vi "LockinFrontPanel.vi"() -> ()   [LabVIEW 2021]
panel:
  in  "?":enum32{"Main", "Phase", "Misc", "Stop"}(tab)
  in  "Set Amplitude":dbl
  in  "Set Amp":bool
  in  "Set Frequency":dbl=1000.0
  in  "Set Freq":bool
  in  "Get Amp":bool
  out "Amplitude":string
  in  "Get Freq":bool
  out "Frequency":string
  in  "Set Sens":bool
  in  "Set Sensitivity":T1(ring)=enum."20 mV"
  in  "Get Sens":bool
  out "Sensitivity":string
  in  "Set TimeC":bool
  in  "Set Time Constant":T2(ring)=enum."10 ms"
  in  "Get TimeC":bool
  out "Time Constant":string
  in  "Autophase":bool
  in  "+90 Phase":bool
  in  "-90 Phase":bool
  in  "Get Phase":bool
  out "Phase":string
  in  "Set Phase":dbl
  in  "Set Ph":bool
  in  "Set A":bool
  in  "Set A-B":bool
  in  "Get Input Setting":bool
  out "A or A-B?":string
  in  "Set Harmonic":i32=1
  in  "Set Harm":bool
  in  "Get Harm":bool
  out "Harmonic":string
  in  "Set Ch 1 Offset":dbl
  in  "Set Offset":bool
  in  "Get Offset":bool
  out "Ch 1 Offset":string
  in  "stop":bool
  # "LOCKIN FRONT PANEL"
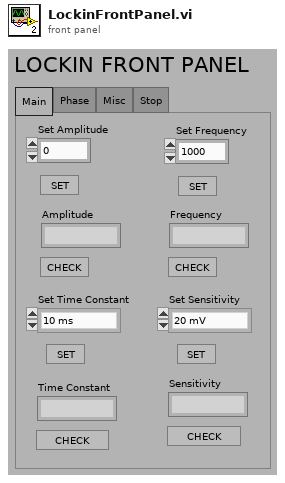
[diagram p1: front panel]
types:
  T1 = enum16{"2 nV", "5 nV", "10 nV", "20 nV", "50 nV", "100 nV", "200 nV", "500 nV", "1 uV", "2 uV", "5 uV", "10 uV", "20 uV", "50 uV", "100 uV", "200 uV", "500 uV", "1 mV", "2 mV", "5 mV", "10 mV", "20 mV", "50 mV", "100 mV", "200 mV", "500 mV", "1 V"}
  T2 = enum16{"10 us", "30 us", "100 us", "300 us", "1 ms", "3 ms", "10 ms", "30 ms", "100 ms", "300 ms", "1 s", "3 s", "10 s", "30 s", "100 s", "300 s", "1 ks", "3 ks", "10 ks", "30 ks"}
  T3 = enum16{"Set Amplitude", "Get Amplitude", "Set Frequency", "Get Frequency", "Set Harmonic", "Get Harmonic", "Set Phase", "Get Phase", "Auto Phase", "Add to Phase", "Autogain", "Set Time Constant", "Get Time Constant", "Set Sensitivity", "Get Sensitivity"}
  T4 = enum16{"Set Amplitude", "Get Amplitude", "Set Frequency", "Get Frequency", "Set Harmonic", "Get Harmonic", "Set Phase", "Get Phase", "Auto Phase", "Add to Phase", "Autogain", "Set Time Constant", "Get Time Constant", "Set Sensitivity", "Get Sensitivity", "Set Input A", "Set Input A-B", "Get Input Setting"}
  T5 = enum16{"Set Amplitude", "Get Amplitude", "Set Frequency", "Get Frequency", "Set Harmonic", "Get Harmonic", "Set Phase", "Get Phase", "Auto Phase", "Add to Phase", "Autogain", "Set Time Constant", "Get Time Constant", "Set Sensitivity", "Get Sensitivity", "Set Input A", "Set Input A-B", "Get Input Setting", "Set Offset", "Get Offset"}
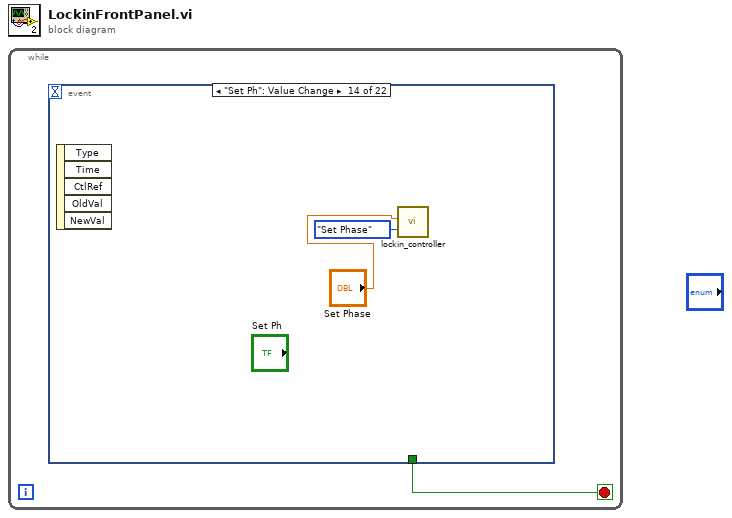
[diagram p0: block diagram]
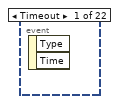
[diagram p2: hidden frame]
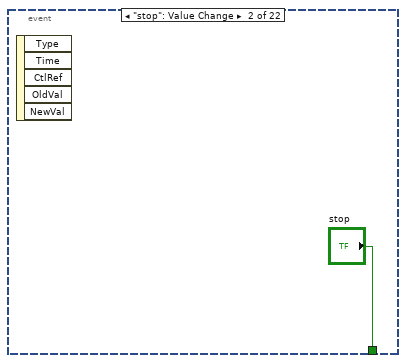
[diagram p3: hidden frame]
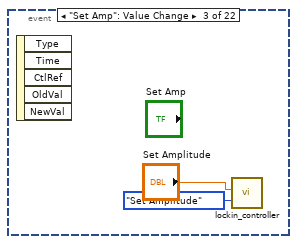
[diagram p4: hidden frame]
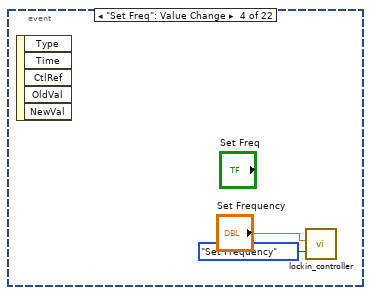
[diagram p5: hidden frame]
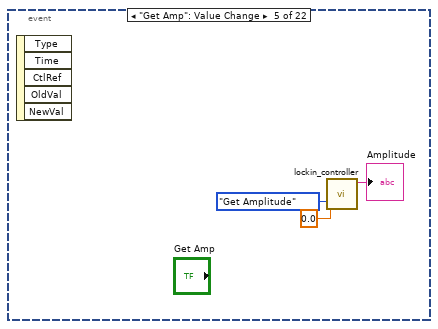
[diagram p6: hidden frame]
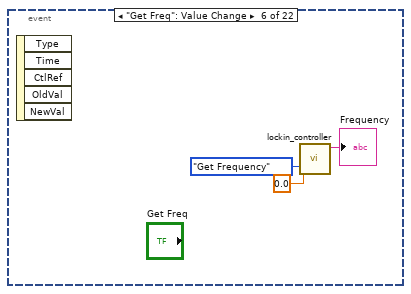
[diagram p7: hidden frame]
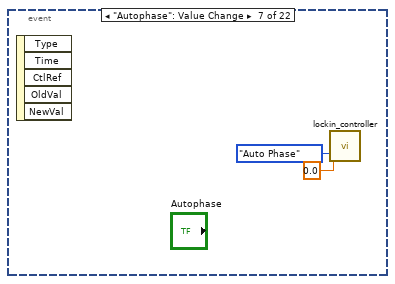
[diagram p8: hidden frame]
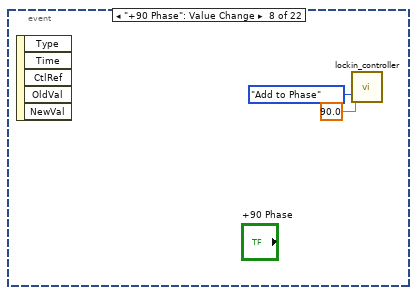
[diagram p9: hidden frame]
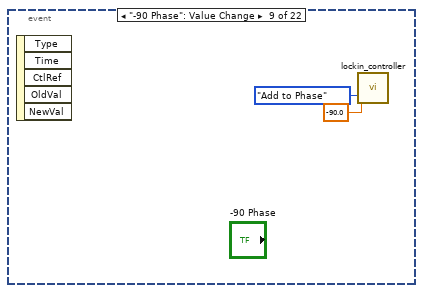
[diagram p10: hidden frame]
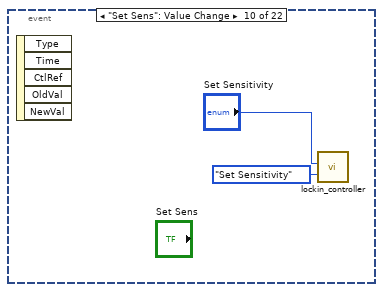
[diagram p11: hidden frame]
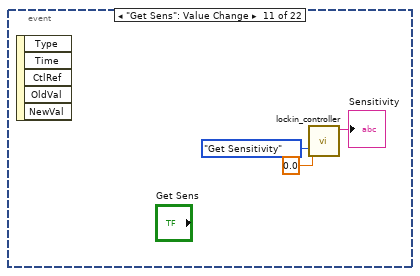
[diagram p12: hidden frame]
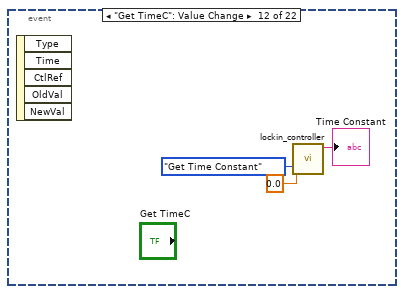
[diagram p13: hidden frame]
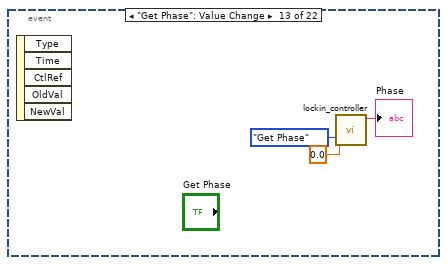
[diagram p14: hidden frame]
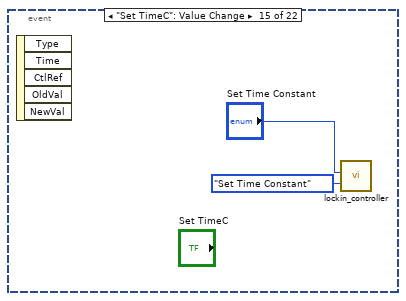
[diagram p15: hidden frame]
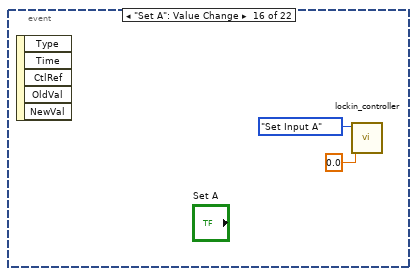
[diagram p16: hidden frame]
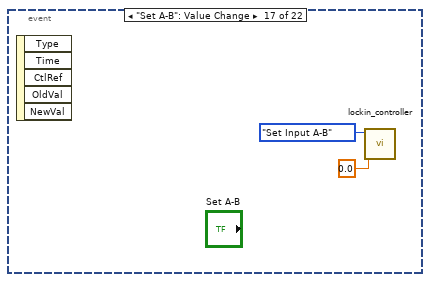
[diagram p17: hidden frame]
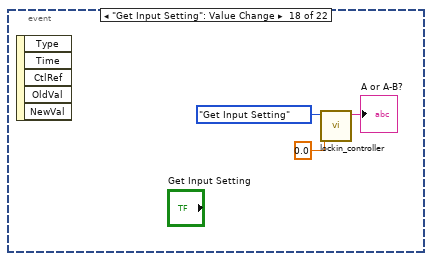
[diagram p18: hidden frame]
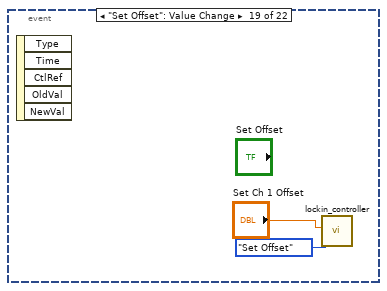
[diagram p19: hidden frame]
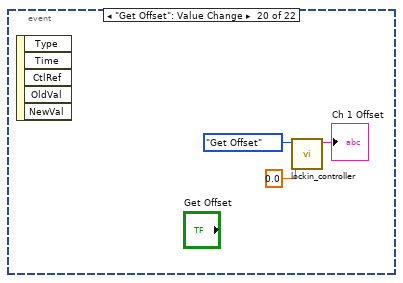
[diagram p20: hidden frame]
diagram:
  n1 = while {
    stop <- w1 stop-if-true
    n2 = event shown="[13] \"Set Ph\": Value Change" {
      selector: _ -> [_ _ _ _ _ _ _ _ _ _ _ _ _ _ _ _ _ _ _ _ _ _]
      dyn-events: _ -> [_ _ _ _ _ _ _ _ _ _ _ _ _ _ _ _ _ _ _ _ _ _]
      timeout: _ -> [_ _ _ _ _ _ _ _ _ _ _ _ _ _ _ _ _ _ _ _ _ _]
      tunnel: [_ "stop" _ _ _ _ _ _ _ _ _ _ _ _ _ _ _ _ _ _ _ _] -> w1
      event Timeout {
        n3 = event-data() -> ()  [unwired: 1 in, 2 out]
      }
      event "stop": Value Change {
        n4 = event-data() -> ()  [unwired: 1 in, 5 out]
      }
      event "Set Amp": Value Change {
        n5 = event-data() -> ()  [unwired: 1 in, 5 out]
        n6 = call "lockin_controller.vi"("Numerical Argument"="Set Amplitude", "Command"=T3."Set Amplitude") -> ()  [unwired: 9 in, 1 out]
      }
      event "Set Freq": Value Change {
        n7 = event-data() -> ()  [unwired: 1 in, 5 out]
        n8 = call "lockin_controller.vi"("Numerical Argument"="Set Frequency", "Command"=T3."Set Frequency") -> ()  [unwired: 9 in, 1 out]
      }
      event "Get Amp": Value Change {
        n9 = event-data() -> ()  [unwired: 1 in, 5 out]
        n10 = call "lockin_controller.vi"("Numerical Argument"=0.0, "Command"=T3."Get Amplitude") -> ("Response"=→"Amplitude":string)  [unwired: 9 in]
      }
      event "Get Freq": Value Change {
        n11 = event-data() -> ()  [unwired: 1 in, 5 out]
        n12 = call "lockin_controller.vi"("Numerical Argument"=0.0, "Command"=T3."Get Frequency") -> ("Response"=→"Frequency":string)  [unwired: 9 in]
      }
      event "Autophase": Value Change {
        n13 = event-data() -> ()  [unwired: 1 in, 5 out]
        n14 = call "lockin_controller.vi"("Numerical Argument"=0.0, "Command"=T3."Auto Phase") -> ()  [unwired: 9 in, 1 out]
      }
      event "+90 Phase": Value Change {
        n15 = event-data() -> ()  [unwired: 1 in, 5 out]
        n16 = call "lockin_controller.vi"("Numerical Argument"=90.0, "Command"=T3."Add to Phase") -> ()  [unwired: 9 in, 1 out]
      }
      event "-90 Phase": Value Change {
        n17 = event-data() -> ()  [unwired: 1 in, 5 out]
        n18 = call "lockin_controller.vi"("Numerical Argument"=-90.0, "Command"=T3."Add to Phase") -> ()  [unwired: 9 in, 1 out]
      }
      event "Set Sens": Value Change {
        n19 = event-data() -> ()  [unwired: 1 in, 5 out]
        n20 = call "lockin_controller.vi"("Numerical Argument"="Set Sensitivity", "Command"=T3."Set Sensitivity") -> ()  [unwired: 9 in, 1 out]
      }
      event "Get Sens": Value Change {
        n21 = event-data() -> ()  [unwired: 1 in, 5 out]
        n22 = call "lockin_controller.vi"("Numerical Argument"=0.0, "Command"=T3."Get Sensitivity") -> ("Response"=→"Sensitivity":string)  [unwired: 9 in]
      }
      event "Get TimeC": Value Change {
        n23 = event-data() -> ()  [unwired: 1 in, 5 out]
        n24 = call "lockin_controller.vi"("Numerical Argument"=0.0, "Command"=T3."Get Time Constant") -> ("Response"=→"Time Constant":string)  [unwired: 9 in]
      }
      event "Get Phase": Value Change {
        n25 = event-data() -> ()  [unwired: 1 in, 5 out]
        n26 = call "lockin_controller.vi"("Numerical Argument"=0.0, "Command"=T3."Get Phase") -> ("Response"=→"Phase":string)  [unwired: 9 in]
      }
      event "Set Ph": Value Change {
        n27 = event-data() -> ()  [unwired: 1 in, 5 out]
        n28 = call "lockin_controller.vi"("Numerical Argument"="Set Phase", "Command"=T3."Set Phase") -> ()  [unwired: 9 in, 1 out]
      }
      event "Set TimeC": Value Change {
        n29 = event-data() -> ()  [unwired: 1 in, 5 out]
        n30 = call "lockin_controller.vi"("Numerical Argument"="Set Time Constant", "Command"=T3."Set Time Constant") -> ()  [unwired: 9 in, 1 out]
      }
      event "Set A": Value Change {
        n31 = event-data() -> ()  [unwired: 1 in, 5 out]
        n32 = call "lockin_controller.vi"("Numerical Argument"=0.0, "Command"=T4."Set Input A") -> ()  [unwired: 9 in, 1 out]
      }
      event "Set A-B": Value Change {
        n33 = event-data() -> ()  [unwired: 1 in, 5 out]
        n34 = call "lockin_controller.vi"("Numerical Argument"=0.0, "Command"=T4."Set Input A-B") -> ()  [unwired: 9 in, 1 out]
      }
      event "Get Input Setting": Value Change {
        n35 = event-data() -> ()  [unwired: 1 in, 5 out]
        n36 = call "lockin_controller.vi"("Numerical Argument"=0.0, "Command"=T4."Get Input Setting") -> ("Response"=→"A or A-B?":string)  [unwired: 9 in]
      }
      event "Set Offset": Value Change {
        n37 = event-data() -> ()  [unwired: 1 in, 5 out]
        n38 = call "lockin_controller.vi"("Numerical Argument"="Set Ch 1 Offset", "Command"=T5."Set Offset") -> ()  [unwired: 9 in, 1 out]
      }
      event "Get Offset": Value Change {
        n39 = event-data() -> ()  [unwired: 1 in, 5 out]
        n40 = call "lockin_controller.vi"("Numerical Argument"=0.0, "Command"=T5."Get Offset") -> ("Response"=→"Ch 1 Offset":string)  [unwired: 9 in]
      }
      event "Set Harm": Value Change {
        n41 = event-data() -> ()  [unwired: 1 in, 5 out]
        n42 = call "lockin_controller.vi"("Numerical Argument"="Set Harmonic", "Command"=T5."Set Harmonic") -> ()  [unwired: 9 in, 1 out]
      }
      event "Get Harm": Value Change {
        n43 = event-data() -> ()  [unwired: 1 in, 5 out]
        n44 = call "lockin_controller.vi"("Numerical Argument"=0.0, "Command"=T5."Get Harmonic") -> ("Response"=→"Harmonic":string)  [unwired: 9 in]
      }
    }
  }
